vi "exp3.vi"() -> ()   [LabVIEW 2022 SP3]
panel:
  in  "实际":bool
  in  "数值 3":i32
  in  "直流偏移":sgl
  in  "采样频率（Hz）":sgl
  in  "初始相位":sgl
  in  "占空比（%）":i8
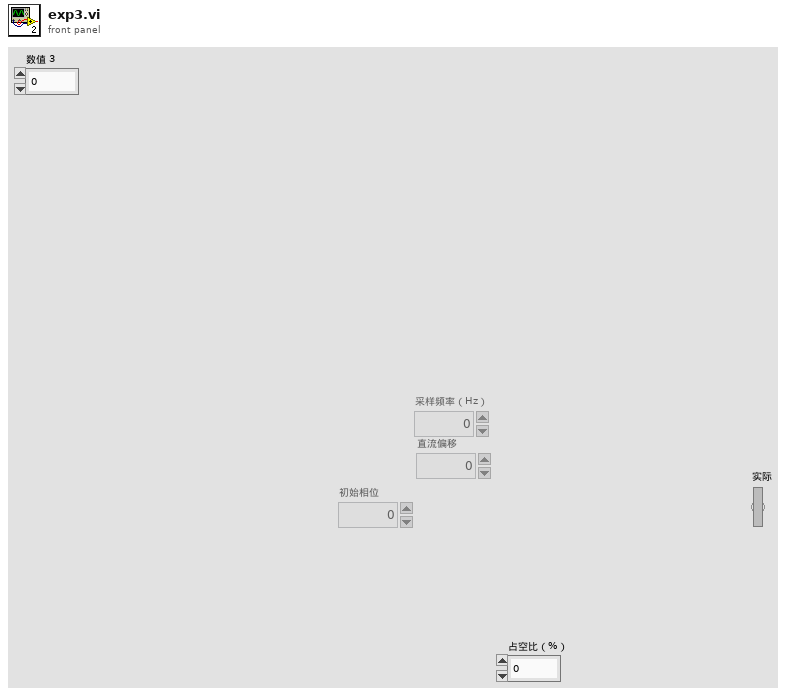
[diagram p1: front panel]
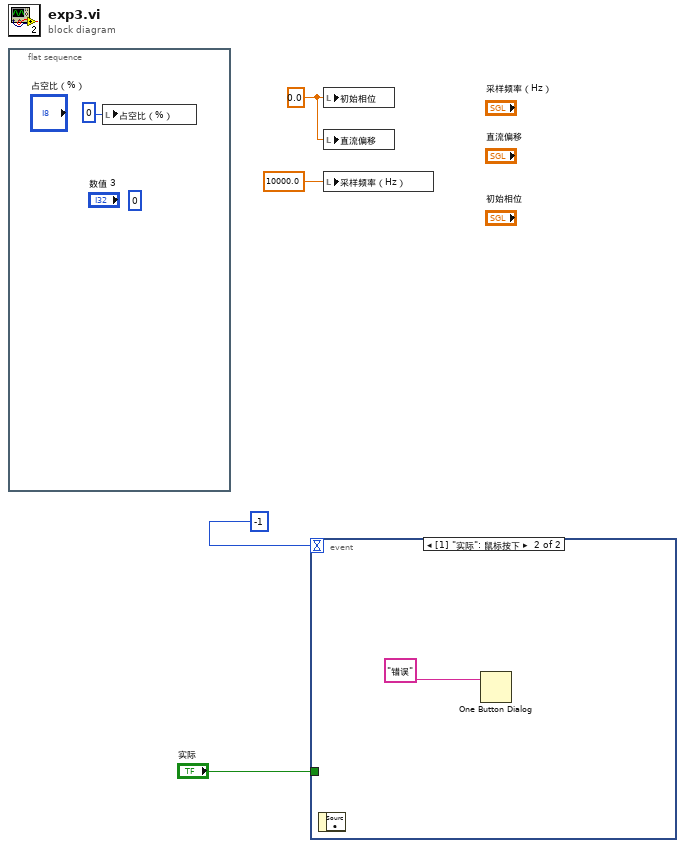
[diagram p0: block diagram]
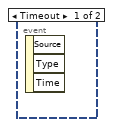
[diagram p2: hidden frame]
diagram:
  w4 = 0.0
  n1 = flat-sequence {
    frame #0 {
      (unwired) 0
      n2 = local write "占空比（%）"(0) -> ()
    }
  }
  n3 = event shown="[1] \"实际\": 鼠标按下" {
    selector: _ -> [_ _]
    dyn-events: _ -> [_ _]
    timeout: -1 -> [_ _]
    tunnel: "实际" -> [_ _]
    event Timeout {
      n4 = event-data() -> ()  [unwired: 1 in, 3 out]
    }
    event "实际": Mouse Down {
      n5 = event-data() -> ()  [unwired: 1 in, 1 out]
      n6 = One Button Dialog(message="错误") -> ()  [unwired: 1 in, 1 out]
    }
  }
  n7 = local write "初始相位"(w4) -> ()
  n8 = local write "直流偏移"(w4) -> ()
  n9 = local write "采样频率（Hz）"(10000.0) -> ()
